vi "DAQ_StopClear.vi"(8 "error in":errorcluster caption="entrée d'erreur") -> (0 "error out":errorcluster caption="sortie d'erreur")   [LabVIEW 2026]
uses:
  Controls/TypeDef_FGV.ctl
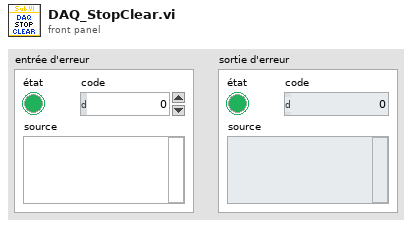
[diagram p1: front panel]
types:
  T1 = typedef "TypeDef_FGV.ctl" = enum16{"Initialize", "Write", "Read"}
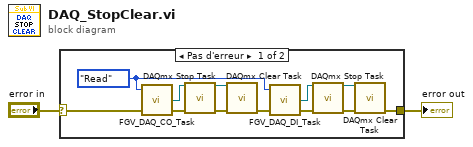
[diagram p0: block diagram]
diagram:
  n1 = case shown="Pas d'erreur" "error in" {
    selector: "error in" -> [w14 w15]
    tunnel: [w4 w15] -> w1
    frame No Error {
      w7 = TypeDef_FGV."Read" ("Action")
      n2 = call "FGV_DAQ_CO_Task.vi"("error in"=w14, "Action"=w7) -> ("error out"=w12:errorcluster, "CO task"=w13:refnum<k21>)  [unwired: 2 in]
      n3 = call <vilib>:"DAQmx Stop Task.vi"("task/channels in"=w13, "error in"=w12) -> ("task out"=w11:refnum<k21>, "error out"=w10:errorcluster)  [unwired: 12 in]
      n4 = call <vilib>:"DAQmx Clear Task.vi"("task in"=w11, "error in"=w10) -> ("error out"=w6:errorcluster)  [unwired: 13 in]
      n5 = call "FGV_DAQ_DI_Task.vi"("error in"=w6, "Action"=w7) -> ("error out"=w3:errorcluster, "DI task"=w5:refnum<k21>)  [unwired: 2 in]
      n6 = call <vilib>:"DAQmx Stop Task.vi"("task/channels in"=w5, "error in"=w3) -> ("task out"=w8:refnum<k21>, "error out"=w9:errorcluster)  [unwired: 12 in]
      n7 = call <vilib>:"DAQmx Clear Task.vi"("task in"=w8, "error in"=w9) -> ("error out"=w4:errorcluster)  [unwired: 13 in]
    }
    frame Error {
    }
  }
  "error out" <- w1
